vi "Lorentzian Function.vi"(3 "output control":T1, 4 "data":variant, 5 "X":dbl[](array[numeric]), 6 "params":dbl[](array[numeric])) -> (0 "error out":errorcluster, 1 "f'(X,a)":dbl[][](array[numeric]), 2 "f(X,a)":dbl[](array[numeric]))   [LabVIEW 2014]
doc: "Given a set of x-values and parameters (x0, gamma), outputs the resulting Lorentzian curve.\n\n(Connector panel is in a form that allows this VI to be passed to the Nonlinear Curve Fit.vi.)"
uses:
  <vilib>/gmath/NumericalOptimization/LM_output select.ctl
  <vilib>/gmath/NI_Gmath.lvlib
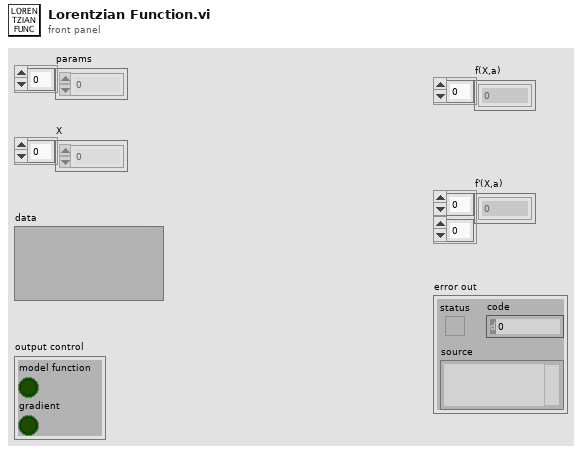
[diagram p1: front panel]
types:
  T1 = typedef "NI_Gmath.lvlib/LM_output select.ctl" = cluster{"model function":bool, "gradient":bool}
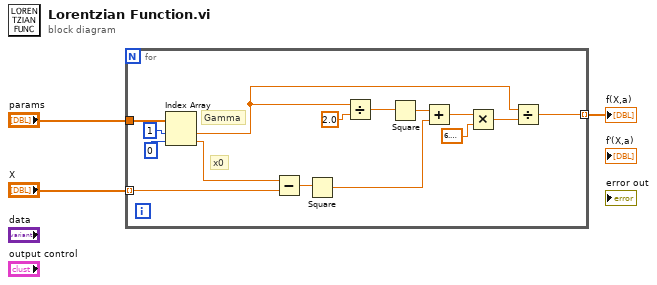
[diagram p0: block diagram]
diagram:
  n1 = for {
    tunnel: "params" -> [w8]
    tunnel: "X" -> [w7] mode=indexing
    tunnel: [w6] -> w1 mode=indexing
    # "x0"
    # "Gamma"
    n2 = Index Array(array=w8, index #1=1 ("index (col)"), index #2=0 ("disabled index (col)")) -> (element #1=w12:dbl, element #2=w13:dbl)
    n3 = Subtract(x=w13, y=w7) -> (x-y=w18:dbl)
    n4 = Square(x=w18) -> (x^2=w14:dbl)
    n5 = Divide(x=w12, y=2.0) -> (x/y=w16:dbl)
    n6 = Square(x=w16) -> (x^2=w15:dbl)
    n7 = Add(x=w15, y=w14) -> (x+y=w11:dbl)
    n8 = Multiply(x=w11, y=6.283185307179586) -> (x*y=w9:dbl)
    n9 = Divide(x=w12, y=w9) -> (x/y=w6:dbl)
  }
  "f(X,a)" <- w1
